vi "subvi_AsciiToWchar.vi"(7 "Text Buffer Size":i32, 10 "ASCII string IN":string) -> (2 "Flattened wchar":string, 5 "Byte Array":u8[](array[numeric]))   [LabVIEW 2013]
doc: "Integral API by Labsphere - DLL wrapper VI\n(c) 2013\n\nTakes LabVIEW ASCII characters in (or empty string if left blank) and creates a bytes-as-text buffer of <b>wchar_t</b> as required by the API. \n\nThis buffer is exactly big enough to hold the number of wchar in \"Text Buffer Size\" in."
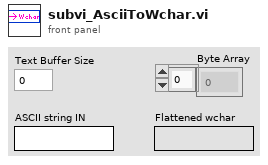
[diagram p1: front panel]
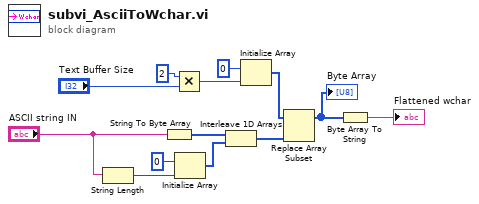
[diagram p0: block diagram]
diagram:
  n1 = String Length(string="ASCII string IN") -> (length=w2:i32)
  n2 = String To Byte Array(string="ASCII string IN") -> (unsigned byte array=w4:u8[])
  n3 = Multiply(x=2, y="Text Buffer Size") -> (x*y=w6:i32)
  n4 = Initialize Array(u8 0, w2) -> (w3:u8[])
  n5 = Interleave 1D Arrays(w4, w3) -> (w11:u8[])
  n6 = Initialize Array(u8 0, w6) -> (w10:u8[])
  n7 = Replace Array Subset(array=w10, new element=w11) -> (w12:u8[])  [unwired: 1 in]
  "Byte Array" <- w12
  n8 = Byte Array To String(unsigned byte array=w12) -> (string=→"Flattened wchar":string)
